vi "Bundle.vi"(8 "error in":errorcluster, 10 "Instrument Info Array":T1[](array[typedef]), 11 "Instrument List Data in":refnum<class "Instrument List Data.lvclass">) -> (0 "error out":errorcluster, 3 "Instrument List Data out":refnum<class "Instrument List Data.lvclass">)   [LabVIEW 2020, in "Instrument Handler.lvlib" / "Instrument List Data.lvclass"]
doc: "Populate the Instrument List Data."
uses:
  Instrument List Data.lvclass
  Controls/Ctl_InstrumentInfo.ctl
  Instrument List Data.lvclass/Instrument List Data.ctl
  Instrument Handler.lvlib
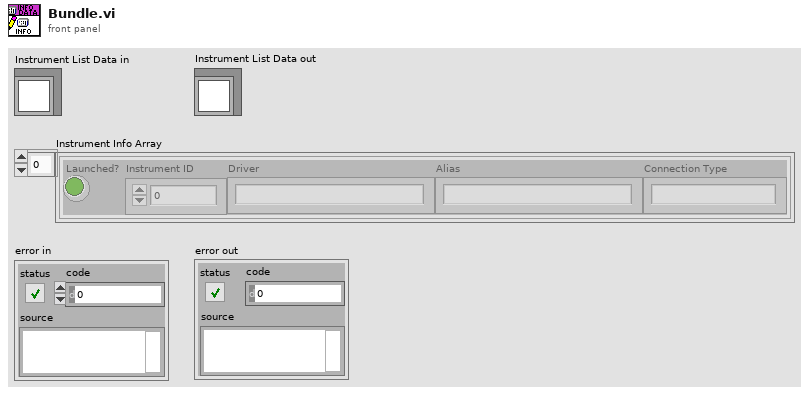
[diagram p1: front panel]
types:
  T1 = typedef "Instrument Handler.lvlib/Ctl_InstrumentInfo.ctl" = cluster{"Launched?":bool, "Instrument ID":u32, "Driver":string, "Alias":string, "Connection Type":string}
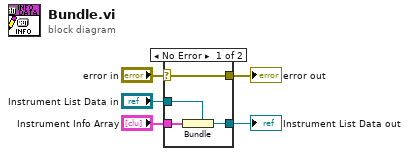
[diagram p0: block diagram]
diagram:
  n1 = case shown="No Error" "error in" {
    selector: "error in" -> [w6 w10]
    tunnel: [w9 w11] -> w5
    tunnel: "Instrument List Data in" -> [w8 w11]
    tunnel: "Instrument Info Array" -> [w7 _]
    tunnel: [w6 w10] -> w1
    frame No Error {
      n2 = Bundle(cluster=w8, w7) -> (w9:refnum<class "Instrument List Data.lvclass">)
    }
    frame Error {
    }
  }
  "Instrument List Data out" <- w5
  "error out" <- w1
